vi "BRig_RT__Case_Idle__State_RewardCalibration_pre__v2.vi"(0 "input_dataMTrig":u16[](array[numeric])) -> (20 "output_dataMTrig":u16[](array[numeric]))   [LabVIEW 2014]
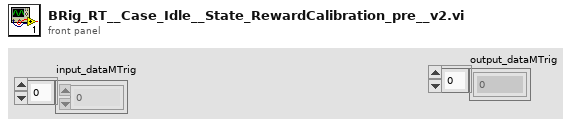
[diagram p1: front panel]
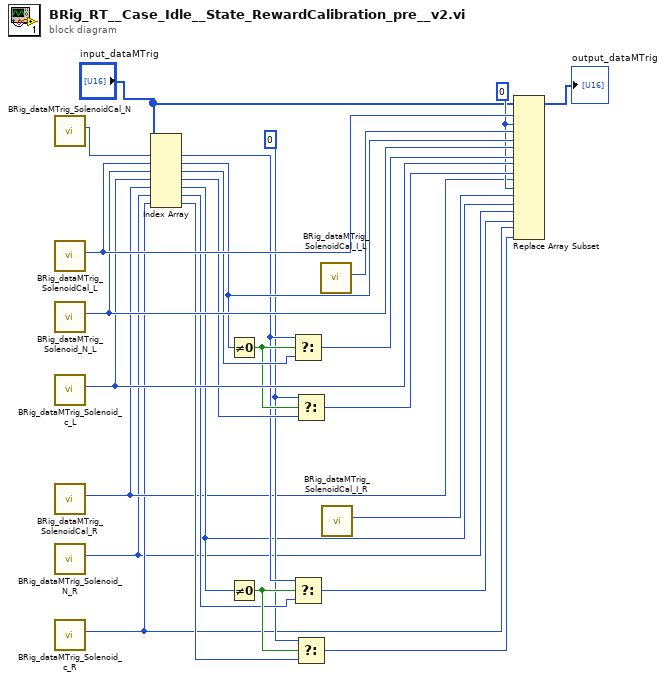
[diagram p0: block diagram]
diagram:
  w12 = u16 0 ("t")
  w6 = u16 0 ("new element/subarray")
  n1 = call "BRig_dataMTrig_SolenoidCal_N.vi"() -> ("output_SolenoidCal_N"=w24:i32)  [unwired: 11 in]
  n2 = call "BRig_dataMTrig_SolenoidCal_L.vi"() -> ("output_SolenoidCal_L"=w26:i32)  [unwired: 11 in]
  n3 = call "BRig_dataMTrig_Solenoid_N_L.vi"() -> ("output_Solenoid_N_L"=w23:i32)  [unwired: 11 in]
  n4 = call "BRig_dataMTrig_Solenoid_c_L.vi"() -> ("output_Solenoid_c_L"=w19:i32)  [unwired: 11 in]
  n5 = call "BRig_dataMTrig_SolenoidCal_R.vi"() -> ("output_SolenoidCal_R"=w5:i32)  [unwired: 11 in]
  n6 = call "BRig_dataMTrig_Solenoid_N_R.vi"() -> ("output_Solenoid_N_R"=w3:i32)  [unwired: 11 in]
  n7 = call "BRig_dataMTrig_Solenoid_c_R.vi"() -> ("output_Solenoid_c_R"=w4:i32)  [unwired: 11 in]
  n8 = Index Array(array="input_dataMTrig", index #1=w24, index #2=w26, index #3=w23, index #4=w19, index #5=w5, index #6=w3, index #7=w4) -> (element #1=w13:u16, element #2=w22:u16, element #3=w21:u16, element #4=w17:u16, element #5=w10:u16, element #6=w15:u16, element #7=w14:u16)
  n9 = Not Equal To 0?(x=w22) -> (x != 0?=w18:bool)
  n10 = Not Equal To 0?(x=w10) -> (x != 0?=w16:bool)
  n11 = Select(t=w13, s=w18, f=w21) -> (s? t:f=w20:u16)
  n12 = Select(t=w13, s=w16, f=w15) -> (s? t:f=w9:u16)
  n13 = Select(t=w12, s=w18, f=w17) -> (s? t:f=w8:u16)
  n14 = Select(t=w12, s=w16, f=w14) -> (s? t:f=w7:u16)
  n15 = call "BRig_dataMTrig_SolenoidCal_I_L.vi"() -> ("output_SolenoidCal_I_L"=w25:i32)  [unwired: 11 in]
  n16 = call "BRig_dataMTrig_SolenoidCal_I_R.vi"() -> ("output_SolenoidCal_I_R"=w11:i32)  [unwired: 11 in]
  n17 = Replace Array Subset(array="input_dataMTrig", new element #1=w6, index #1=w26, new element #2=w22, index #2=w25, new element #3=w20, index #3=w23, new element #4=w8, index #4=w19, new element #5=w6, index #5=w5, new element #6=w10, index #6=w11, new element #7=w9, index #7=w3, new element #8=w7, index #8=w4) -> (→"output_dataMTrig":u16[])
